vi "EEPROM cmd send, wait for ACK.vi"(4 "Slot":u8 max=7, 6 "Error In":errorcluster, 7 "Single slot EEPROM values":T1[](array[typedef])=[{"Pmin (Pa)"=0.0, "Pmax (Pa)"=0.0, "maxCount"=0, "minCount"=0, "Poffset (Pa)"=0.0}, {"Pmin (Pa)"=0.0, "Pmax (Pa)"=0.0, "maxCount"=0, "minCount"=0, "Poffset (Pa)"=0.0}, {"Pmin (Pa)"=0.0, "Pmax (Pa)"=0.0, "maxCount"=0, "minCount"=0, "Poffset (Pa)"=0.0}, {"Pmin (Pa)"=0.0, "Pmax (Pa)"=0.0, "maxCount"=0, "minCount"=0, "Poffset (Pa)"=0.0}, {"Pmin (Pa)"=0.0, "Pmax (Pa)"=0.0, "maxCount"=0, "minCount"=0, "Poffset (Pa)"=0.0}, {"Pmin (Pa)"=0.0, "Pmax (Pa)"=0.0, "maxCount"=0, "minCount"=0, "Poffset (Pa)"=0.0}, {"Pmin (Pa)"=0.0, "Pmax (Pa)"=0.0, "maxCount"=0, "minCount"=0, "Poffset (Pa)"=0.0}, {"Pmin (Pa)"=0.0, "Pmax (Pa)"=0.0, "maxCount"=0, "minCount"=0, "Poffset (Pa)"=0.0}], 8 "R / W":string(combo)="R", 9 "VISA resource name in":refnum<visa-resource-name>) -> (0 "Error out":errorcluster, 1 "Single slot EEPROM values returned":T1[](array[typedef]), 2 "ACK ok":bool, 3 "VISA resource name out":refnum<visa-resource-name>)   [LabVIEW 2015]
uses:
  Ctls/EEPROM page.ctl
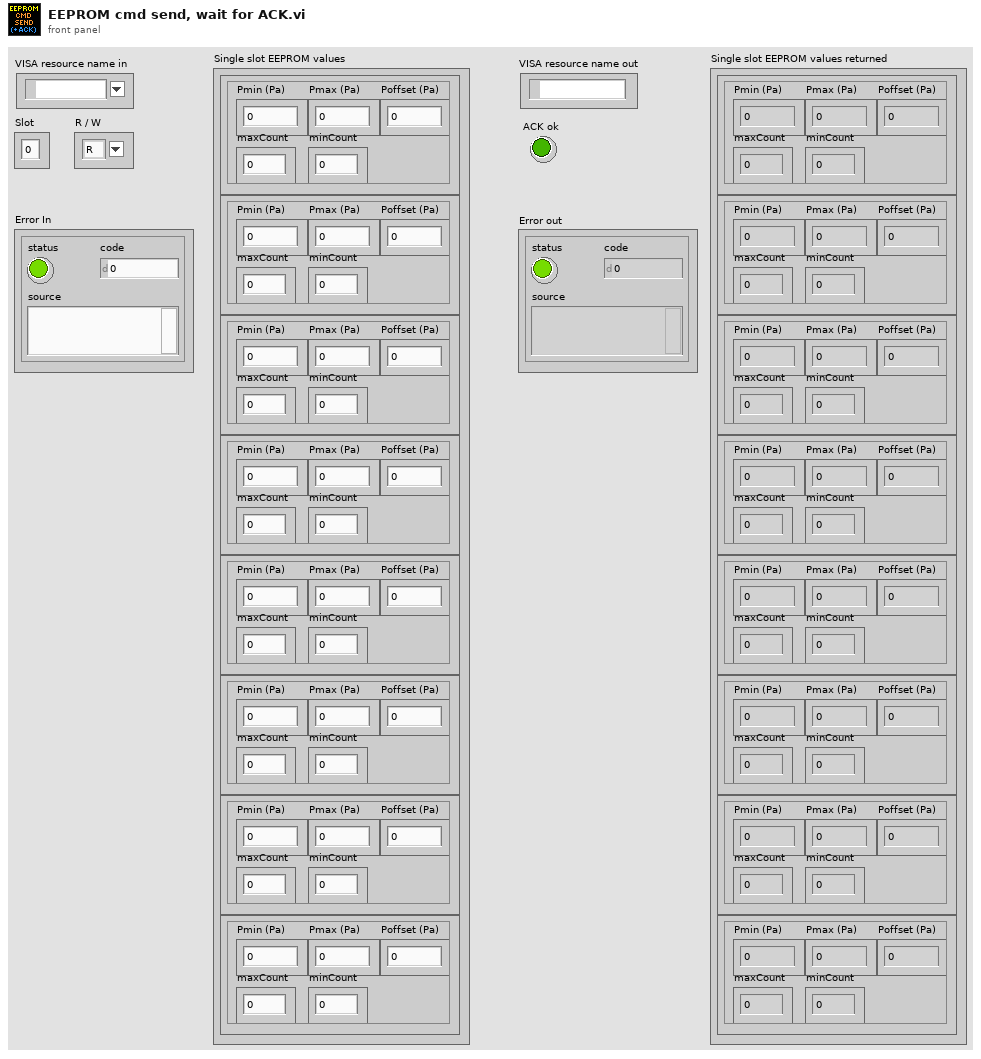
[diagram p1: front panel]
types:
  T1 = typedef "EEPROM page.ctl" = cluster{"Pmin (Pa)":sgl, "Pmax (Pa)":sgl, "maxCount":u16, "minCount":u16, "Poffset (Pa)":sgl}
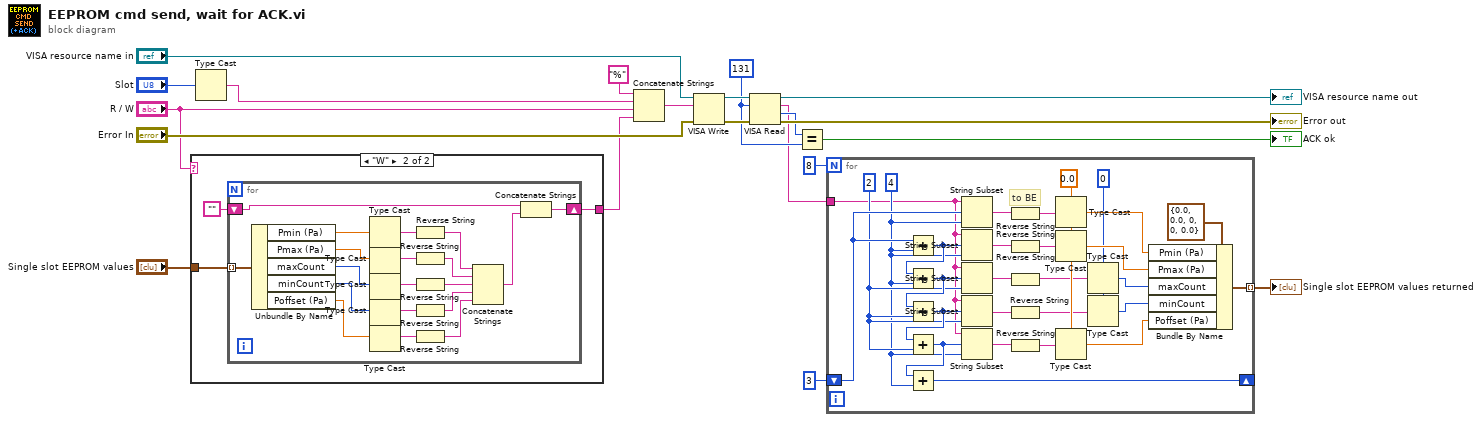
[diagram p0: block diagram]
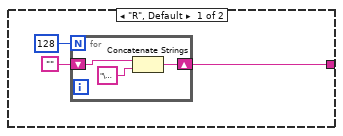
[diagram p2: hidden frame]
diagram:
  w10 = u32 131 ("byte count")
  n1 = case shown="\"W\"" "R / W" {
    tunnel: "Single slot EEPROM values" -> [_ w29]
    tunnel: [w22 w27] -> w7
    frame "R", Default {
      n2 = for {
        N: 128 -> [_]
        shift-right: [w25] -> w22
        shift-left: "" -> [w24]
        n3 = Concatenate Strings(w24, "\u0000") -> (w25:string)
      }
    }
    frame "W" {
      n4 = for {
        tunnel: w29 -> [w48] mode=indexing
        shift-right: [w31] -> w27
        shift-left: "" -> [w30]
        n5 = Unbundle By Name(w48) -> ("Pmin (Pa)"=w47:sgl, "Pmax (Pa)"=w41:sgl, "maxCount"=w40:u16, "minCount"=w39:u16, "Poffset (Pa)"=w38:sgl)
        n6 = Type Cast(x=w47) -> (*(type *) &x=w46:string)  [unwired: 1 in]
        n7 = Type Cast(x=w41) -> (*(type *) &x=w45:string)  [unwired: 1 in]
        n8 = Type Cast(x=w40) -> (*(type *) &x=w44:string)  [unwired: 1 in]
        n9 = Type Cast(x=w39) -> (*(type *) &x=w43:string)  [unwired: 1 in]
        n10 = Type Cast(x=w38) -> (*(type *) &x=w42:string)  [unwired: 1 in]
        n11 = Reverse String(1:w46) -> (0:w37:string)
        n12 = Reverse String(1:w45) -> (0:w36:string)
        n13 = Reverse String(1:w44) -> (0:w35:string)
        n14 = Reverse String(1:w43) -> (0:w34:string)
        n15 = Reverse String(1:w42) -> (0:w33:string)
        n16 = Concatenate Strings(w37, w36, w35, w34, w33) -> (w32:string)
        n17 = Concatenate Strings(w30, w32) -> (w31:string)
      }
    }
  }
  n18 = Type Cast(x="Slot") -> (*(type *) &x=w5:string)  [unwired: 1 in]
  n19 = Concatenate Strings("%" ("string"), w5, "R / W", w7) -> (w12:string)
  n20 = VISA Write(VISA resource name="VISA resource name in", write buffer=w12, error in (no error)="Error In") -> (VISA resource name out=w18:refnum<visa-resource-name>, error out=w16:errorcluster)  [unwired: 1 out]
  n21 = VISA Read(VISA resource name=w18, byte count=w10, error in (no error)=w16) -> (VISA resource name out=→"VISA resource name out":refnum<visa-resource-name>, read buffer=w1:string, return count=w11:u32, error out=→"Error out":errorcluster)
  n22 = Equal?(x=w11, y=w10) -> (x = y?=→"ACK ok":bool)
  n23 = for {
    N: 8 -> [_]
    shift-right: [w68] -> _
    shift-left: 3 ("offset (0)") -> [w75]
    tunnel: [w60] -> w2 mode=indexing
    tunnel: w1 -> [w59]
    w71 = 2 ("length (rest)")
    w69 = 4 ("length (rest)")
    w63 = u16 0
    w76 = sgl 0.0
    # "to BE"
    n24 = Add(x=w75, y=w69) -> (x+y=w74:i32)
    n25 = Add(x=w74, y=w69) -> (x+y=w73:i32)
    n26 = Add(x=w73, y=w71) -> (x+y=w72:i32)
    n27 = Add(x=w72, y=w71) -> (x+y=w70:i32)
    n28 = Add(x=w70, y=w69) -> (x+y=w68:i32)
    n29 = String Subset(string=w59, offset (0)=w75, length (rest)=w69) -> (substring=w58:string)
    n30 = String Subset(string=w59, offset (0)=w74, length (rest)=w69) -> (substring=w55:string)
    n31 = String Subset(string=w59, offset (0)=w73, length (rest)=w71) -> (substring=w54:string)
    n32 = String Subset(string=w59, offset (0)=w72, length (rest)=w71) -> (substring=w53:string)
    n33 = String Subset(string=w59, offset (0)=w70, length (rest)=w69) -> (substring=w52:string)
    n34 = Reverse String(1:w58) -> (0:w57:string)
    n35 = Reverse String(1:w55) -> (0:w56:string)
    n36 = Reverse String(1:w54) -> (0:w49:string)
    n37 = Reverse String(1:w53) -> (0:w50:string)
    n38 = Reverse String(1:w52) -> (0:w51:string)
    n39 = Type Cast(type=w76, x=w57) -> (*(type *) &x=w66:sgl)
    n40 = Type Cast(type=w76, x=w56) -> (*(type *) &x=w65:sgl)
    n41 = Type Cast(type=w76, x=w51) -> (*(type *) &x=w61:sgl)
    n42 = Type Cast(type=w63, x=w49) -> (*(type *) &x=w64:u16)
    n43 = Type Cast(type=w63, x=w50) -> (*(type *) &x=w62:u16)
    n44 = Bundle By Name(cluster=T1 {"Pmin (Pa)"=0.0, "Pmax (Pa)"=0.0, "maxCount"=0, "minCount"=0, "Poffset (Pa)"=0.0} ("Page"), "Pmin (Pa)"=w66, "Pmax (Pa)"=w65, "maxCount"=w64, "minCount"=w62, "Poffset (Pa)"=w61) -> (w60:T1)
  }
  "Single slot EEPROM values returned" <- w2
